vi "Function.vi"(8 "error in (no error)":errorcluster, 10 "Value":sgl, 11 "Two Terminal in":refnum<class "Increment_SGL.lvclass">) -> (0 "error out":errorcluster, 2 "Result":sgl, 3 "Two Terminal out":refnum<class "Increment_SGL.lvclass">)   [LabVIEW 2021, in "Increment_SGL.lvclass"]
uses:
  Increment_SGL.lvclass
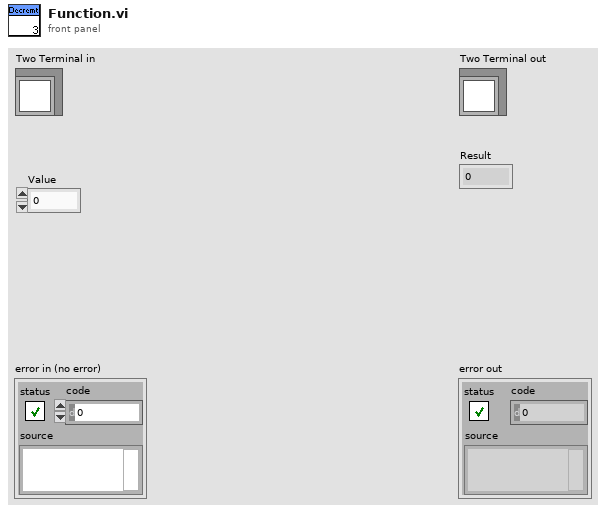
[diagram p1: front panel]
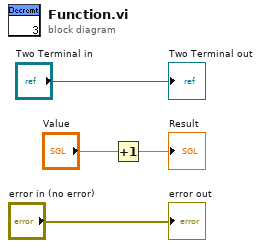
[diagram p0: block diagram]
diagram:
  n1 = Increment(x="Value") -> (x+1=→"Result":sgl)
  "error out" <- "error in (no error)"
  "Two Terminal out" <- "Two Terminal in"
